vi "Get Temperature.vi"(6 "Channel":i32, 8 "error in (no error)":errorcluster, 11 "instrument.PPMS in":refnum<class "instrument.PPMS1.lvclass">) -> (0 "error out":errorcluster, 1 "Status":variant, 2 "Temperature (K)":dbl, 3 "instrument.PPMS out":refnum<class "instrument.PPMS1.lvclass">, 4 "Finished?":bool)   [LabVIEW 2019, in "instrument.PPMS1.lvclass"]
uses:
  instrument.PPMS1.lvclass
  instrument.PPMS/Typedefs/PPMS.Temperature Status--cluster.ctl
  instrument.PPMS/instrument.PPMS.lvclass
  Typedefs/PPMS1.Commands-enum.ctl
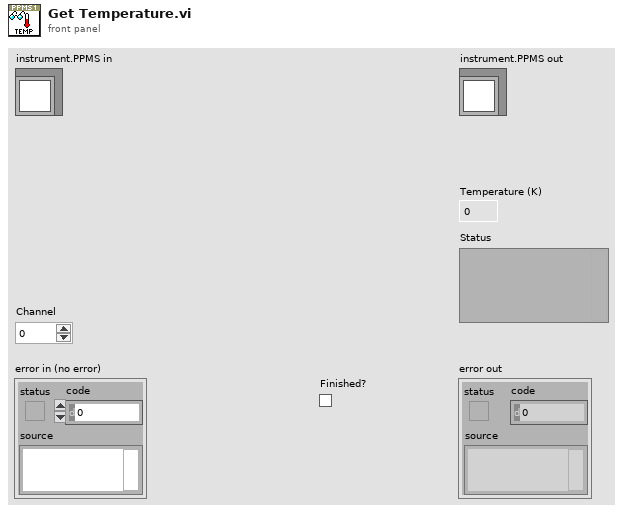
[diagram p1: front panel]
types:
  T1 = typedef "instrument.PPMS1.lvclass/PPMS1.Commands-enum.ctl" = enum16{"Get Magnet Field", "Get Helium Level", "Get Temperature", "Set Magnet Field", "Set Temperature", "getAll"}
  T2 = typedef "instrument.PPMS.lvclass/PPMS.Temperature Status--cluster.ctl" = cluster{"Temperature (K)":dbl, "Temperature Status":string}
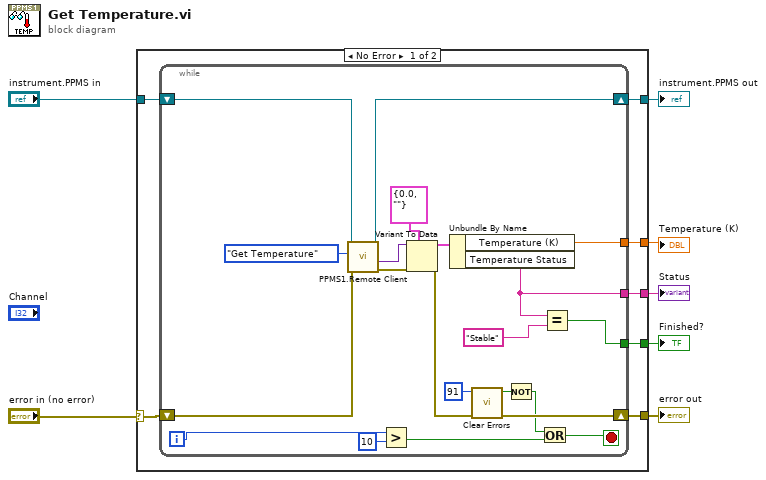
[diagram p0: block diagram]
diagram:
  n1 = case shown="No Error" "error in (no error)" {
    selector: "error in (no error)" -> [w10 w37]
    tunnel: [w14 _] -> w7
    tunnel: [w9 w37] -> w6
    tunnel: [w13 w36] -> w5
    tunnel: "instrument.PPMS in" -> [w12 w36]
    tunnel: [w11 _] -> w3
    tunnel: [w8 _] -> w1
    frame No Error {
      n2 = while {
        tunnel: [w35] -> w14
        tunnel: [w17] -> w11
        shift-right: [w33] -> w13
        shift-left: w12 -> [w32]
        shift-right: [w26] -> w9
        shift-left: w10 -> [w27]
        tunnel: [w15] -> w8
        i -> [w21]
        stop <- w20 stop-if-true
        n3 = call "PPMS1.Remote Client.vi"("error in (no error)"=w27, "Command"=PPMS1.Commands-enum."Get Temperature", "instrument.PPMS1 in"=w32) -> ("error out"=w29:errorcluster, "Data out"=w28:variant, "instrument.PPMS1 out"=w33:refnum<class "instrument.PPMS1.lvclass">)  [unwired: 5 in, 1 out]
        n4 = Greater?(x=w21, y=10) -> (0:w22:bool)
        n5 = Variant To Data(error in=w29, type=T2 {"Temperature (K)"=0.0, "Temperature Status"=""} ("Temperature Status"), Variant=w28) -> (data=w30:T2, error out=w34:errorcluster)
        n6 = Unbundle By Name(w30) -> ("Temperature (K)"=w35:dbl, "Temperature Status"=w17:string)
        n7 = call <vilib>:"Clear Errors.vi"("error in (no error)"=w34, "specific error code to clear (0: all)"=91) -> ("error out"=w26:errorcluster, "specific error cleared?"=w19:bool)  [unwired: 4 in]
        n8 = Not(x=w19) -> (.not. x?=w18:bool)
        n9 = Or(x=w18, y=w22) -> (x .or. y?=w20:bool)
        n10 = Equal?(x=w17, y="Stable" ("Temperature Status")) -> (x = y?=w15:bool)
      }
    }
    frame Error {
    }
  }
  "error out" <- w6
  "instrument.PPMS out" <- w5
  "Temperature (K)" <- w7
  "Status" <- w3
  "Finished?" <- w1
